vi "Process Active Data Shift Key.vi"(7 "# User Layers":i32, 9 "VKey":T1, 11 "Active Data [] in":i32[](array[numeric])) -> (3 "Active Data [] out":i32[](array[numeric]))   [LabVIEW 2020]
uses:
  <vilib>/event_ctls.llb/eventvkey.ctl
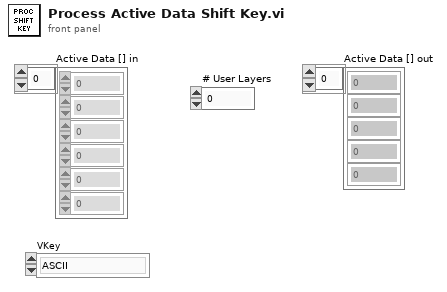
[diagram p1: front panel]
types:
  T1 = typedef "eventvkey.ctl" = enum16{"ASCII", "Enter", "Return", "Shift", "Ctrl", "Alt", "Cmd", "Opt", "Caps", "NumLock", "Clear", "Break", "Up", "Down", "Left", "Right", "Insert", "Delete", "Home", "End", "PageUp", "PageDown", "Escape", "Help", "Pause", "ScrollLock", "F1", "F2", "F3", "F4", "F5", "F6", "F7", "F8", "F9", "F10", "F11", "F12", "F13", "F14", "F15", "F16", "F17", "F18", "F19", "F20", "F21", "F22", "F23", "F24", "Play", "VolumeUp", "VolumeDown", "Mute", "Two Byte Char"}
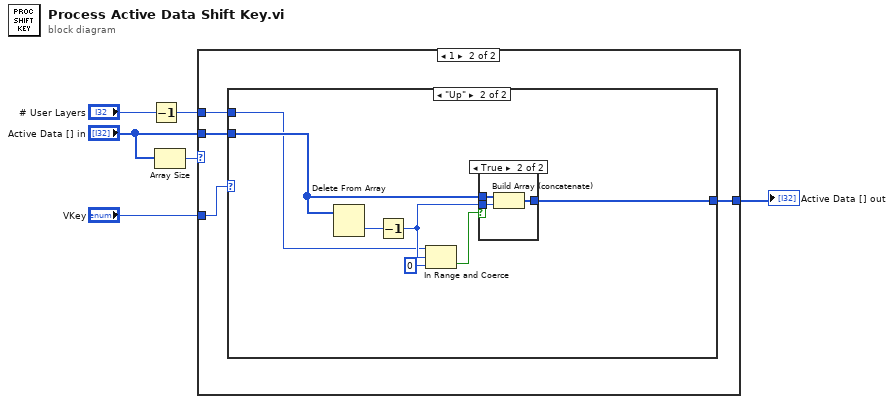
[diagram p0: block diagram]
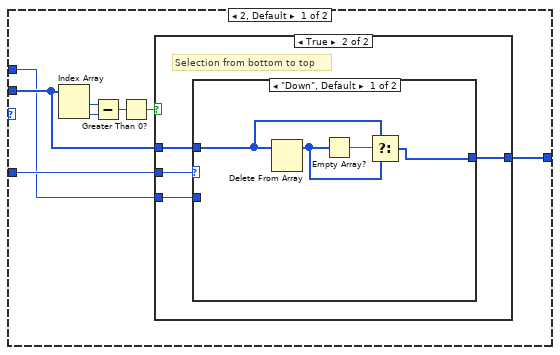
[diagram p2: hidden frame]
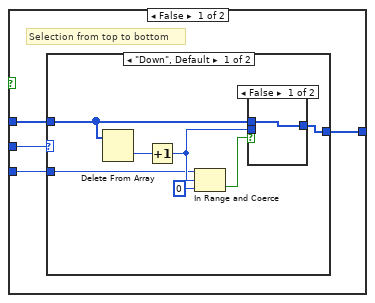
[diagram p3: hidden frame]
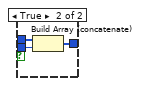
[diagram p4: hidden frame]
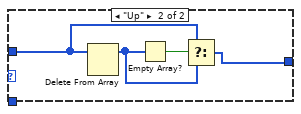
[diagram p5: hidden frame]
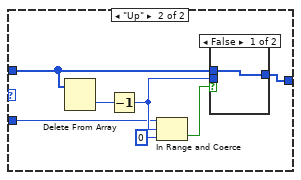
[diagram p6: hidden frame]
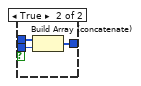
[diagram p7: hidden frame]
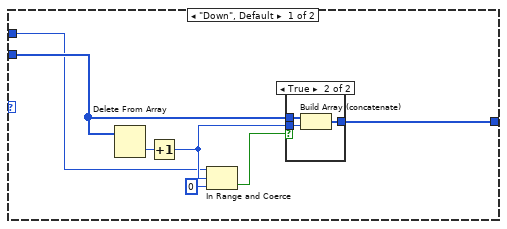
[diagram p8: hidden frame]
diagram:
  n1 = Decrement(x="# User Layers") -> (x-1=w5:i32)
  n2 = Array Size(array="Active Data [] in") -> (size(s)=w1:i32)
  n3 = case shown="1" w1 {
    tunnel: "VKey" -> [w10 w56]
    tunnel: "Active Data [] in" -> [w9 w55]
    tunnel: w5 -> [w7 w54]
    tunnel: [w8 w53] -> w6
    frame 2, Default {
      n4 = Index Array(array=w9) -> (element #1=w13:i32, element #2=w14:i32)  [unwired: 2 in]
      n5 = Subtract(x=w13, y=w14) -> (x-y=w12:i32)
      n6 = Greater Than 0?(x=w12) -> (x > 0?=w11:bool)
      n7 = case shown="True" w11 {
        tunnel: w10 -> [w18 w37]
        tunnel: w9 -> [w17 w36]
        tunnel: [w16 w35] -> w8
        tunnel: w7 -> [w15 w34]
        frame False {
          # "Selection from top to bottom"
          n8 = case shown="\"Down\", Default" w18 {
            tunnel: w17 -> [w20 w31]
            tunnel: [w21 w30] -> w16
            tunnel: w15 -> [w19 _]
            frame "Down", Default {
              n9 = Delete From Array(array=w20) -> (deleted portion=w25:i32)  [unwired: 2 in, 1 out]
              n10 = Increment(x=w25) -> (x+1=w24:i32)
              n11 = In Range and Coerce(upper limit=w19, x=w24, lower limit=0) -> (In Range?=w22:bool)  [unwired: 1 out]
              n12 = case shown="False" w22 {
                tunnel: w20 -> [w26 w29]
                tunnel: [w26 w28] -> w21
                tunnel: w24 -> [_ w27]
                frame False {
                }
                frame True {
                  n13 = Build Array (concatenate)(w29, w27) -> (w28:i32[])
                }
              }
            }
            frame "Up" {
              n14 = Delete From Array(array=w31) -> (array with subset deleted=w32:i32[])  [unwired: 2 in, 1 out]
              n15 = Empty Array?(array=w32) -> (empty?=w33:bool)
              n16 = Select(t=w31, s=w33, f=w32) -> (s? t:f=w30:i32[])
            }
          }
        }
        frame True {
          # "Selection from bottom to top"
          n17 = case shown="\"Down\", Default" w37 {
            tunnel: w36 -> [w39 w43]
            tunnel: [w38 w44] -> w35
            tunnel: w34 -> [_ w42]
            frame "Down", Default {
              n18 = Delete From Array(array=w39) -> (array with subset deleted=w40:i32[])  [unwired: 2 in, 1 out]
              n19 = Empty Array?(array=w40) -> (empty?=w41:bool)
              n20 = Select(t=w39, s=w41, f=w40) -> (s? t:f=w38:i32[])
            }
            frame "Up" {
              n21 = Delete From Array(array=w43) -> (deleted portion=w48:i32)  [unwired: 2 in, 1 out]
              n22 = Decrement(x=w48) -> (x-1=w47:i32)
              n23 = In Range and Coerce(upper limit=w42, x=w47, lower limit=0) -> (In Range?=w45:bool)  [unwired: 1 out]
              n24 = case shown="False" w45 {
                tunnel: w43 -> [w49 w52]
                tunnel: [w49 w51] -> w44
                tunnel: w47 -> [_ w50]
                frame False {
                }
                frame True {
                  n25 = Build Array (concatenate)(w52, w50) -> (w51:i32[])
                }
              }
            }
          }
        }
      }
    }
    frame 1 {
      n26 = case shown="\"Up\"" w56 {
        tunnel: w55 -> [w63 w74]
        tunnel: w54 -> [w60 w71]
        tunnel: [w57 w68] -> w53
        frame "Down", Default {
          n27 = Delete From Array(array=w63) -> (deleted portion=w62:i32)  [unwired: 2 in, 1 out]
          n28 = Increment(x=w62) -> (x+1=w61:i32)
          n29 = In Range and Coerce(upper limit=w60, x=w61, lower limit=0) -> (In Range?=w58:bool)  [unwired: 1 out]
          n30 = case shown="True" w58 {
            tunnel: w63 -> [w64 w67]
            tunnel: [w64 w66] -> w57
            tunnel: w61 -> [_ w65]
            frame False {
            }
            frame True {
              n31 = Build Array (concatenate)(w67, w65) -> (w66:i32[])
            }
          }
        }
        frame "Up" {
          n32 = Delete From Array(array=w74) -> (deleted portion=w73:i32)  [unwired: 2 in, 1 out]
          n33 = Decrement(x=w73) -> (x-1=w72:i32)
          n34 = In Range and Coerce(upper limit=w71, x=w72, lower limit=0) -> (In Range?=w69:bool)  [unwired: 1 out]
          n35 = case shown="True" w69 {
            tunnel: w74 -> [w75 w78]
            tunnel: [w75 w77] -> w68
            tunnel: w72 -> [_ w76]
            frame False {
            }
            frame True {
              n36 = Build Array (concatenate)(w78, w76) -> (w77:i32[])
            }
          }
        }
      }
    }
  }
  "Active Data [] out" <- w6
